vi "RegisterMat_Array1D-CXT.vi"(8 "error in":errorcluster, 11 "Array in":cxt[](array[numeric])) -> (0 "error out":errorcluster, 3 "Image":u8, 4 "AdressOrData":cxt[](array[numeric]), 6 "Mat":T1)   [LabVIEW 2020, in "OpenLvVision_OpenCv.lvlib"]
doc: "Register mat for dll.\nNo malleable to breake vi inlining!"
uses:
  OpenLvVision_OpenCv.lvlib
  TypeDef/MatInfo.ctl
  TypeDef/LvDatatype.ctl
  <vilib>/Utility/error.llb/Error Cluster From Error Code.vi
  <vilib>/ErrorRing/Error Ring.xnode
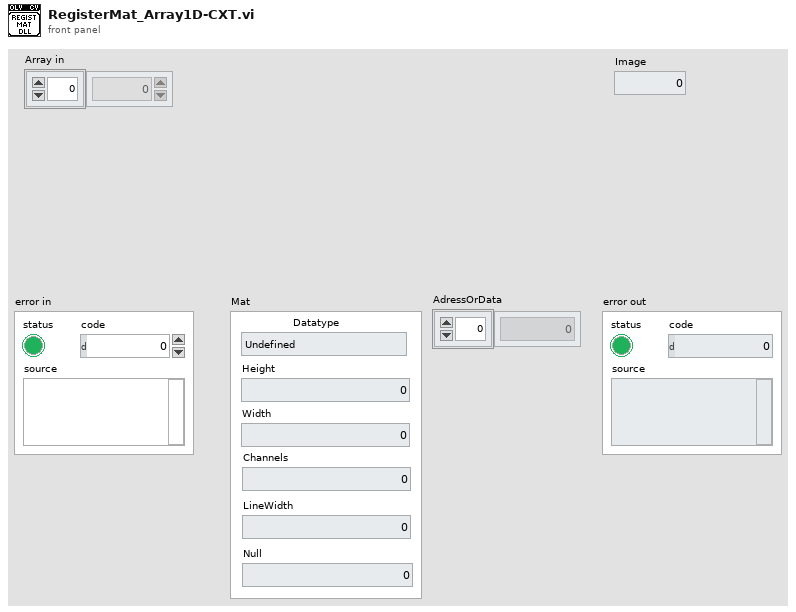
[diagram p1: front panel]
types:
  T1 = typedef "OpenLvVision_OpenCv.lvlib/MatInfo.ctl" = cluster{"Datatype":T2, "Height":i32, "Width":i32, "Channels":i32, "LineWidth":i32, "Null":u8}
  T2 = typedef "OpenLvVision_OpenCv.lvlib/LvDatatype.ctl" = enum32{"Undefined", "U8", "I8", "U16", "I16", "U32_Color", "I32", "U64_Color", "I64", "SGL", "DBL", "Complex SGL", "Complex DBL", "Array 1D U8", "Array 1D I8", "Array 1D U16", "Array 1D I16", "Array 1D U32_Color", "Array 1D I32", "Array 1D U64_Color", "Array 1D I64", "Array 1D SGL", "Array 1D DBL", "Array 1D Complex SGL", "Array 1D Complex DBL", "Array 2D U8", "Array 2D I8", "Array 2D U16", "Array 2D I16", "Array 2D U32", "Array 2D U32_Color", "Array 2D I32", "Array 2D U64", "Array 2D U64_Color", "Array 2D I64", "Array 2D SGL", "Array 2D DBL", "Array 2D Complex SGL", "Array 2D Complex DBL", "Array 3D U8", "Array 3D I8", "Array 3D U16", "Array 3D I16", "Array 3D U32", "Array 3D I32", "Array 3D U64", "Array 3D I64", "Array 3D SGL", "Array 3D DBL", "Array 3D Complex SGL", "Array 3D Complex DBL", "Image Mono U8", "Image Mono U16", "Image Mono I16", "Image Mono SGL", "Image Color U32", "Image Color U64", "ImageComplex Sgl"}
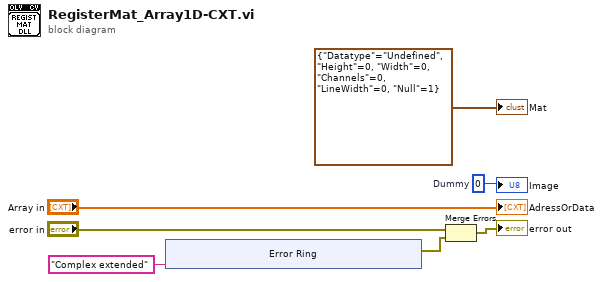
[diagram p0: block diagram]
diagram:
  w7 = u8 0  # Dummy
  n1 = xnode "Error Ring"("parameter 0"="Complex extended") -> ("error out"=w1:errorcluster)
  n2 = Merge Errors("error in", w1) -> (→"error out":errorcluster)
  "Mat" <- T1 {"Datatype"=enum."Undefined", "Height"=0, "Width"=0, "Channels"=0, "LineWidth"=0, "Null"=1} ("LvData")
  "AdressOrData" <- "Array in"
  "Image" <- w7
